vi "Test app for Autocad.vi"() -> ()   [LabVIEW 2015]
uses:
  AutoCAD cmds.ctl
  AguaClara Library.lvlib
  MathCAD results ref.ctl
panel:
  in  "error in (no error)":errorcluster
  out "error out":errorcluster
  in  "path":path=path "C:/Documents and Settings/mw24/My Documents/Drawing2.dwg"
  in  "MathCAD results":T1
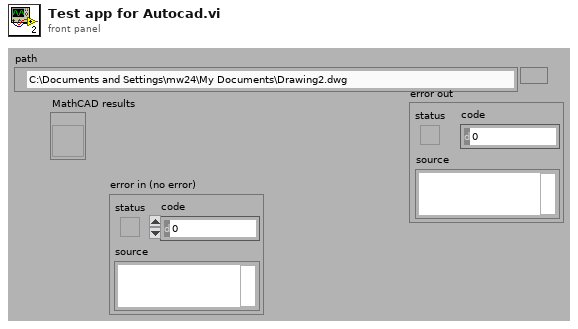
[diagram p1: front panel]
types:
  T1 = typedef "MathCAD results ref.ctl" = refnum<vi>
  T2 = typedef "AguaClara Library.lvlib/AutoCAD cmds.ctl" = enum16{"Open AutoCAD", "New Document", "Send Command", "Send Command Array", "Close Doc", "Quit"}
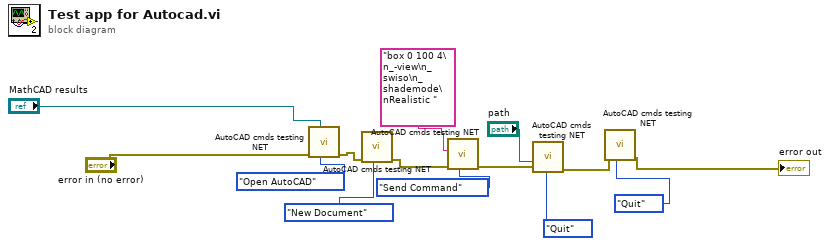
[diagram p0: block diagram]
diagram:
  n1 = call "AutoCAD cmds testing NET.vi"("AutoCAD cmd"=AutoCAD_cmds."Open AutoCAD", "MathCAD results"="MathCAD results", "error in (no error)"="error in (no error)") -> ("error out"=w14:errorcluster)  [unwired: 7 in, 1 out]
  n2 = call "AutoCAD cmds testing NET.vi"("AutoCAD cmd"=AutoCAD_cmds."New Document", "error in (no error)"=w14) -> ("error out"=w8:errorcluster)  [unwired: 8 in, 1 out]
  n3 = call "AutoCAD cmds testing NET.vi"("AutoCAD cmd"=AutoCAD_cmds."Send Command", "error in (no error)"=w8, "Command"="box 0 100 4\n_-view\n_swiso\n_shademode\nRealistic ") -> ("error out"=w9:errorcluster)  [unwired: 7 in, 1 out]
  n4 = call "AutoCAD cmds testing NET.vi"("AutoCAD cmd"=AutoCAD_cmds."Quit", "error in (no error)"=w9, "path"="path") -> ("error out"=w3:errorcluster)  [unwired: 7 in, 1 out]
  n5 = call "AutoCAD cmds testing NET.vi"("AutoCAD cmd"=AutoCAD_cmds."Quit", "error in (no error)"=w3) -> ("error out"=→"error out":errorcluster)  [unwired: 8 in, 1 out]
